vi "joystick experiment.vi"() -> ()   [LabVIEW 2017]
uses:
  <vilib>/Utility/inputDevices.llb/joystickAcquire.vi
  <vilib>/Utility/inputDevices.llb/closeJoystick.vi
panel:
  out "button info":T1
  out "direction info":T2
  out "error out":errorcluster
  out "V-Axis":i32(graph)
  out "Y Rotation":i32(graph)
  out "X Rotation":i32(graph)
  out "Z-Axis":dbl(graph)
  out "Y-Axis":i32(graph)
  out "X-Axis":i32(graph)
  in  "device index":i32
  in  "stop":bool
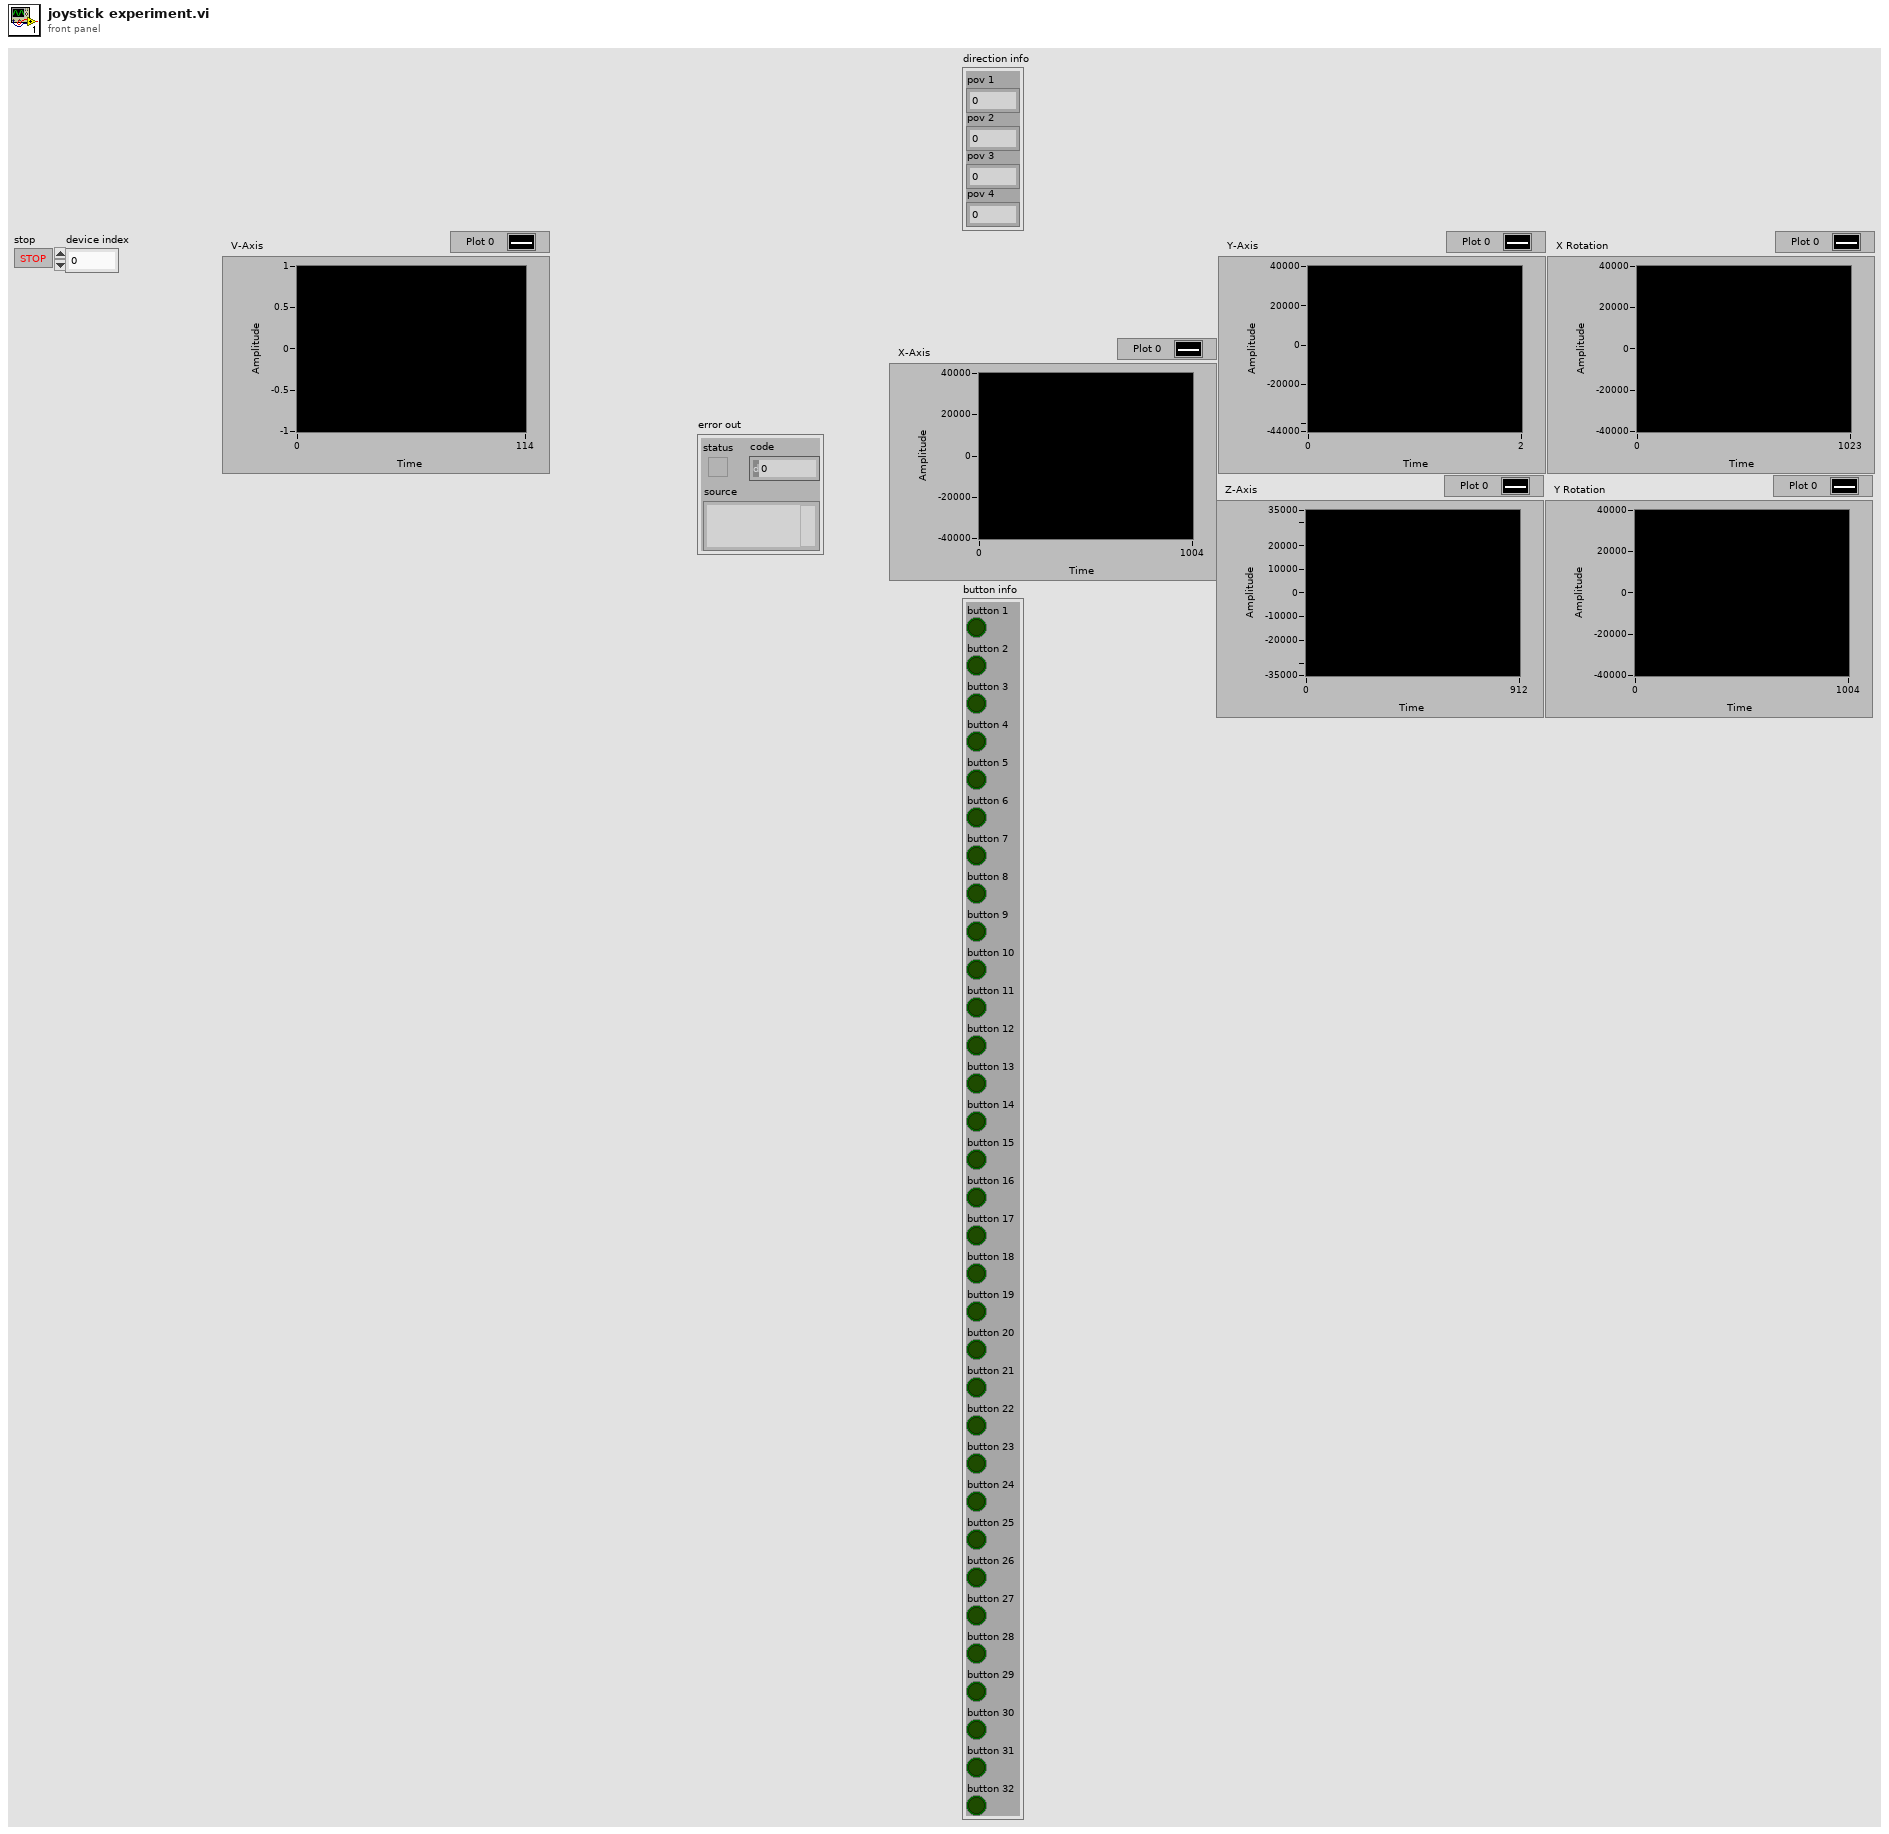
[diagram p1: front panel]
types:
  T1 = cluster{"button 1":bool, "button 2":bool, "button 3":bool, "button 4":bool, "button 5":bool, "button 6":bool, "button 7":bool, "button 8":bool, "button 9":bool, "button 10":bool, "button 11":bool, "button 12":bool, "button 13":bool, "button 14":bool, "button 15":bool, "button 16":bool, "button 17":bool, "button 18":bool, "button 19":bool, "button 20":bool, "button 21":bool, "button 22":bool, "button 23":bool, "button 24":bool, "button 25":bool, "button 26":bool, "button 27":bool, "button 28":bool, "button 29":bool, "button 30":bool, "button 31":bool, "button 32":bool}
  T2 = cluster{"pov 1":i32, "pov 2":i32, "pov 3":i32, "pov 4":i32}
  T3 = cluster{"X axis":i32, "Y axis":i32, "Z axis":i32, "X axis rotation":i32, "Y axis rotation":i32, "Z axis rotation":i32, "U axis":i32, "V axis":i32}
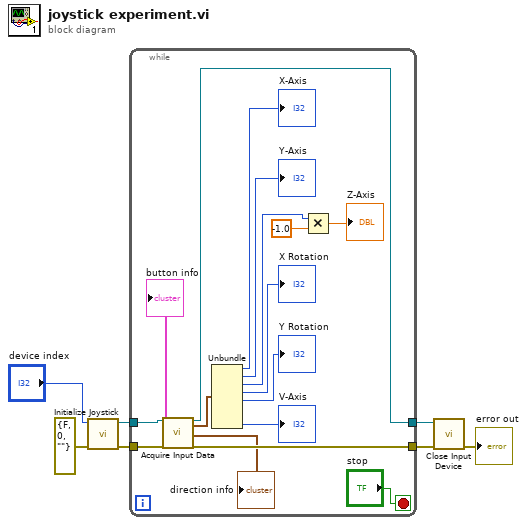
[diagram p0: block diagram]
diagram:
  n1 = call <vilib>:"Initialize Joystick.vi"("error in (no error)"=errorcluster {"status"=FALSE, "code"=0, "source"=""}, "device index"="device index") -> ("error out"=w5:errorcluster, "device ID"=w6:refnum<k1>)  [unwired: 8 in]
  n2 = while {
    tunnel: w6 -> [w22]
    tunnel: w5 -> [w21]
    tunnel: [w16] -> w3
    tunnel: [w15] -> w2
    stop <- "stop" stop-if-true
    n3 = call-poly <vilib>:"Acquire Input Data.vi"("device ID"=w22, "error in (no error)"=w21) -> ("device ID"=w16:refnum<k1>, "axis info"=w20:T3, "button info"=→"button info":T1, "direction info"=→"direction info":T2, "error out"=w15:errorcluster)  [unwired: 13 in]
    n4 = Unbundle(w20) -> ("X axis"=→"X-Axis":i32, "Y axis"=→"Y-Axis":i32, "Z axis"=w10:i32, "X axis rotation"=→"X Rotation":i32, "Y axis rotation"=→"Y Rotation":i32, "V axis"=→"V-Axis":i32)  [unwired: 2 out]
    n5 = Multiply(x=w10, y=-1.0) -> (x*y=→"Z-Axis":dbl)
  }
  n6 = call-poly <vilib>:"Close Input Device.vi"("error in (no error)"=w2, "device ID"=w3) -> ("error out"=→"error out":errorcluster)  [unwired: 8 in]
